vi "GetDataSetProps.vi"(6 "do not write to database":bool, 8 "error in (no error)":errorcluster, 10 "waveform":waveform(sgl), 11 "dataset props in":T1[](array[typedef])) -> (0 "error out":errorcluster, 3 "dataset props out":T1[](array[typedef]))   [LabVIEW 2017, in "DataEventCreator.lvlib"]
uses:
  <vilib>/addons/InsightCM/Devices/Shared/Common/DataEventCreator/DataEventCreator.lvlib
  <vilib>/addons/InsightCM/MessageBus/Base/controls/KeyValuePair.ctl
  <vilib>/addons/InsightCM/Utilities/ChannelStatus/ChannelStatus.lvlib
  <vilib>/addons/InsightCM/Utilities/PropertyHelpers/PropertyHelpers.lvlib
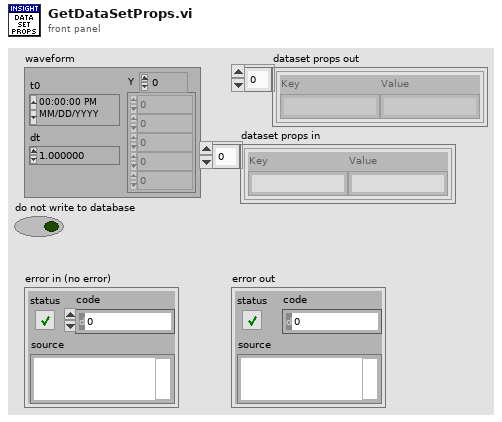
[diagram p1: front panel]
types:
  T1 = typedef "KeyValuePair.ctl" = cluster{"Key":string, "Value":string}
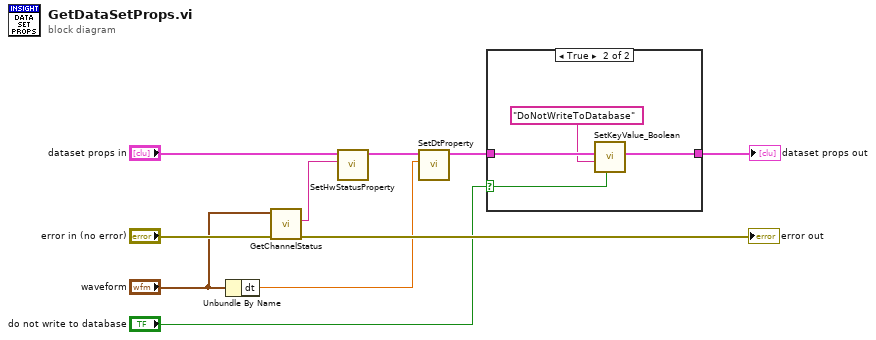
[diagram p0: block diagram]
diagram:
  n1 = Unbundle By Name("waveform") -> ("dt"=w7:dbl)
  n2 = call <vilib>:"GetChannelStatus.vi"("error in (no error)"="error in (no error)", "waveform in"="waveform") -> ("error out"=→"error out":errorcluster, "channel status"=w5:string)  [unwired: 6 in, 2 out]
  n3 = call <vilib>:"SetHwStatusProperty.vi"("hw status"=w5, "props in"="dataset props in") -> ("props out"=w1:T1[])  [unwired: 9 in]
  n4 = call <vilib>:"SetDtProperty.vi"("dt"=w7, "props in"=w1) -> ("props out"=w4:T1[])  [unwired: 9 in]
  n5 = case shown="True" "do not write to database" {
    selector: "do not write to database" -> [_ w12]
    tunnel: w4 -> [w11 w15]
    tunnel: [w11 w14] -> w3
    frame False {
    }
    frame True {
      n6 = call <vilib>:"SetKeyValue_Boolean.vi"("value"=w12, "key"="DoNotWriteToDatabase", "key value pairs"=w15) -> ("key value pairs out"=w14:T1[])  [unwired: 8 in]
    }
  }
  "dataset props out" <- w3
